vi "PrototypeV2_control.vi"() -> ()   [LabVIEW 2019]
uses:
  00d467ad-0018-435b-b1c4-002e486b128f.vi
  2e8d34c2-00e2-46f1-99d0-d57288b70d8f.vi
  0f690846-c94a-4028-9fe1-d10e28cf598c.vi
  4854abb9-ccb6-456c-8c0d-1df9cc9317d1.vi
  <vilib>/Instr/_visa.llb/VISA Configure Serial Port (Instr).vi
  globals.vi
  <vilib>/Utility/file.llb/Read Delimited Spreadsheet (DBL).vi
panel:
  in  "Control SAS":bool
  in  "Control ELO":bool
  in  "UVP OVP BAT2":bool=TRUE
  in  "UVP OVP BAT1":bool=TRUE
  in  "ELO file":path=path "C:/repositories/bdc_controller/hex_logger/source_code/0.5A.csv"
  in  "ELO VISA":refnum<visa-resource-name>="USB0::0x0B3E::0x1019::YL002399::INSTR"
  in  "Orbits":i32=4
  out "Orbital period (s)":dbl
  out "elapsed time":dbl
  in  "SAS file":path=path "C:/repositories/bdc_controller/hex_logger/source_code/SAS_off.csv"
  in  "SAS VISA":refnum<visa-resource-name>="USB0::0x0957::0x1107::MY54001612::INSTR"
  out "CONV2":cluster{u16, u16, i16}(graph)
  out "converter2 file":path
  out "controller file":path
  out "converter1 file":path
  in  "CONVERTER 2 PORT":refnum<visa-resource-name>="COM5"
  out "sync":bool
  in  "CONVERTER 1 PORT":refnum<visa-resource-name>="COM4"
  out "sync":bool
  out "CONV1":cluster{u16, u16, i16}(graph)
  out "3.3V REG":cluster{u16, u16}(graph)
  out "5V REG":cluster{u16, u16}(graph)
  out "BUS":cluster{u16, u16, u16}(graph)
  in  "project name":string
  in  "CONTROL":bool
  in  "CONTROLLER PORT":refnum<visa-resource-name>="COM3"
  out "sync":bool
  in  "STOP":bool
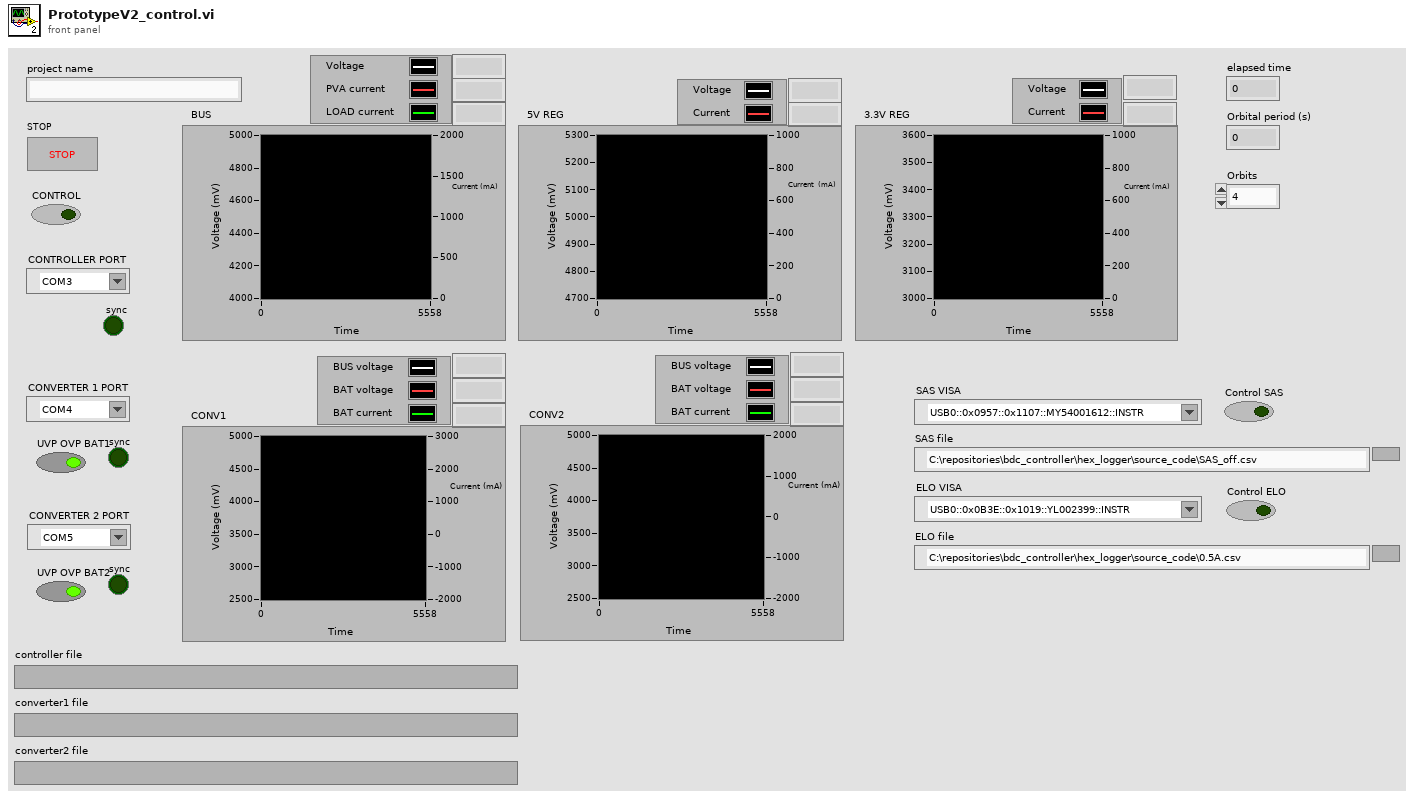
[diagram p1: front panel]
types:
  T1 = cluster{u16, u16, u16, u16, u16, u16, u16, u16, u16}
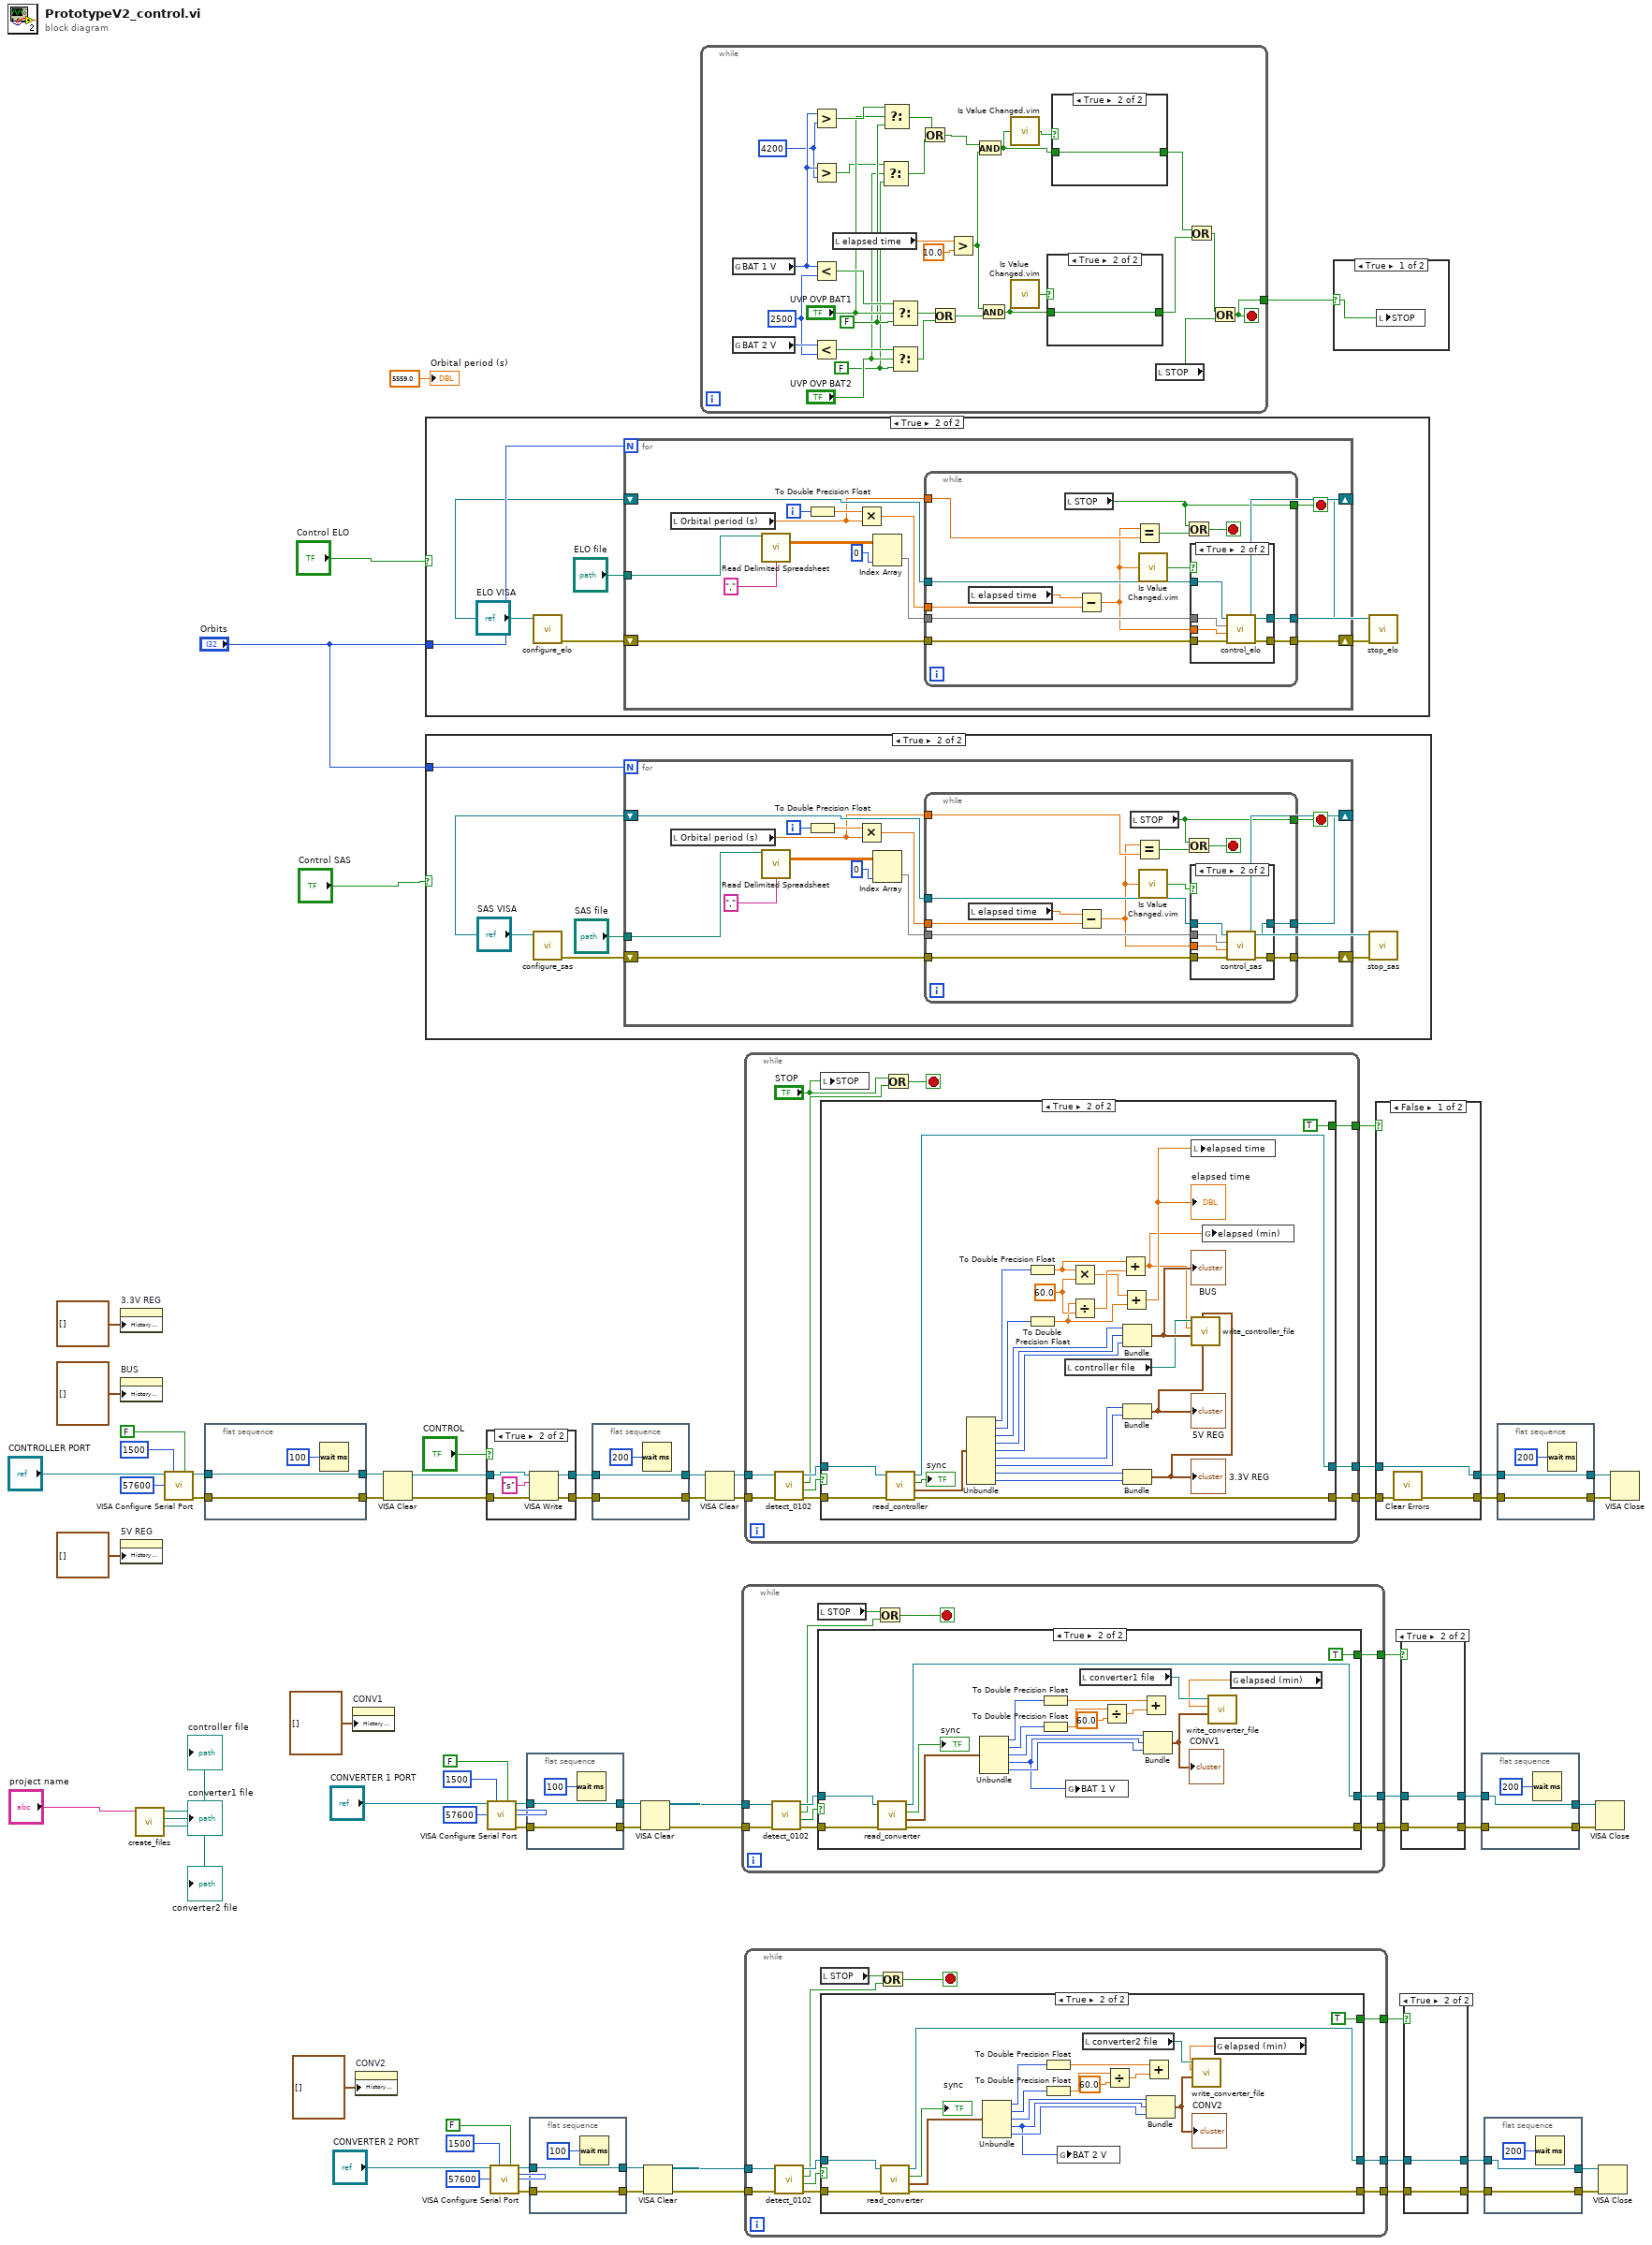
[diagram p0: block diagram]
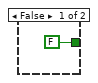
[diagram p7: hidden frame]
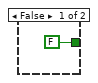
[diagram p8: hidden frame]
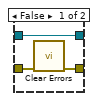
[diagram p9: hidden frame]
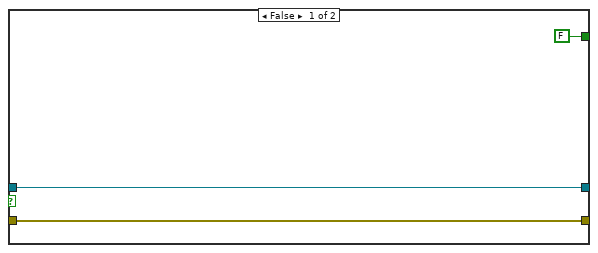
[diagram p10: hidden frame]
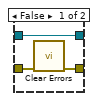
[diagram p11: hidden frame]
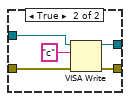
[diagram p12: hidden frame]
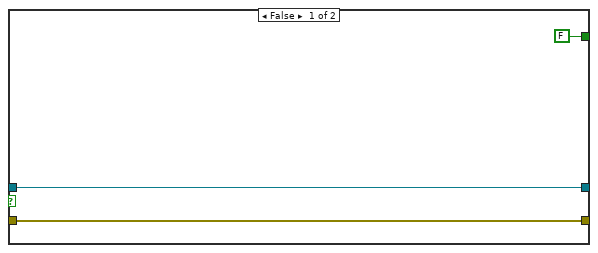
[diagram p13: hidden frame]
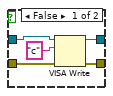
[diagram p14: hidden frame]
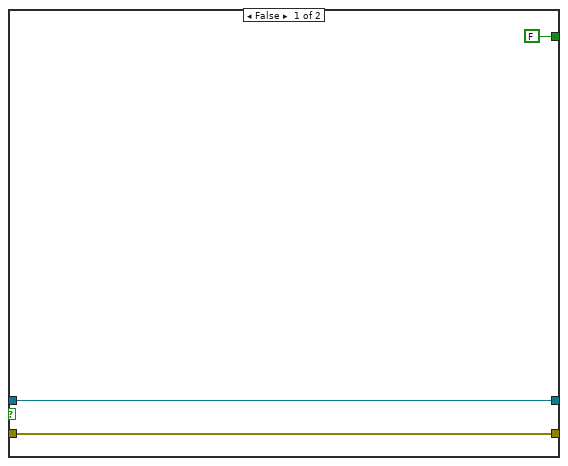
[diagram p15: hidden frame]
diagram:
  n1 = property on="3.3V REG" class="WFChart (strict)"("History Data"=cluster{dbl, dbl}[] []) -> ()  [unwired: 2 in, 2 out]
  n2 = property on="BUS" class="WFChart (strict)"("History Data"=cluster{dbl, dbl, dbl}[] []) -> ()  [unwired: 2 in, 2 out]
  n3 = property on="5V REG" class="WFChart (strict)"("History Data"=cluster{dbl, dbl}[] []) -> ()  [unwired: 2 in, 2 out]
  n4 = call "create_files.vi"("project name"="project name") -> ("converter2"=→"converter2 file":path, "converter1"=→"converter1 file":path, "controller"=→"controller file":path)  [unwired: 8 in]
  n5 = call-poly "VISA Configure Serial Port"("VISA resource name"="CONTROLLER PORT", "timeout (10sec)"=u32 1500, "Enable Termination\nChar (T)"=FALSE ("Enable Termination\nChar (T)"), "baud rate (9600)"=u32 57600) -> ("VISA resource name out"=w69:refnum<visa-resource-name>, "error out"=w68:errorcluster)  [unwired: 10 in]
  n6 = flat-sequence {
    tunnel: w68 -> [w74]
    tunnel: [w74] -> w67
    tunnel: [w73] -> w66
    tunnel: w69 -> [w73]
    frame #0 {
      n7 = Wait (ms)(milliseconds to wait=u32 100) -> ()  [unwired: 1 out]
    }
  }
  n8 = property on="CONV1" class="WFChart (strict)"("History Data"=cluster{dbl, dbl, dbl}[] []) -> ()  [unwired: 2 in, 2 out]
  n9 = property on="CONV2" class="WFChart (strict)"("History Data"=cluster{dbl, dbl, dbl}[] []) -> ()  [unwired: 2 in, 2 out]
  n10 = VISA Clear(VISA resource name=w66, error in (no error)=w67) -> (VISA resource name out=w65:refnum<visa-resource-name>, error out=w64:errorcluster)
  n11 = case shown="True" "Control ELO" {
    tunnel: "Orbits" -> [_ w81]
    frame False {
    }
    frame True {
      n12 = call "configure_elo.vi"("VISA Refnum in"="ELO VISA") -> ("error out"=w78:errorcluster, "VISA Refnum out"=w79:refnum<visa-resource-name>)  [unwired: 8 in, 1 out]
      n13 = for {
        N: w81 -> [_]
        shift-right: [w94] -> w77
        shift-left: w79 -> [w96]
        shift-right: [w93] -> w76
        shift-left: w78 -> [w95]
        tunnel: "ELO file" -> [w85]
        i -> [w91]
        stop <- w83 stop-if-true
        n14 = local read "Orbital period (s)"() -> (w89:dbl)
        n15 = call-poly <vilib>:"Read Delimited Spreadsheet.vi"("file path (dialog if empty)"=w85, "delimiter (\\t)"="," ("delimiter (\\t)")) -> ("all rows"=w88:dbl[][])  [unwired: 8 in, 5 out]
        n16 = To Double Precision Float(number=w91) -> (double precision float=w92:dbl)
        n17 = Multiply(x=w92, y=w89) -> (x*y=w90:dbl)
        n18 = Index Array(array=w88, index (col)=0 ("disabled index (col)")) -> (element=w84:dbl[])  [unwired: 1 in]
        n19 = while {
          tunnel: w96 -> [w109]
          tunnel: w95 -> [w108]
          tunnel: w84 -> [w107]
          tunnel: [w105] -> w94
          tunnel: [w104] -> w93
          tunnel: w90 -> [w103]
          tunnel: w89 -> [w101]
          tunnel: [w97] -> w83
          stop <- w98 stop-if-true
          n20 = local read "elapsed time"() -> (w102:dbl)
          n21 = local read "STOP"() -> (w97:bool)
          n22 = Subtract(x=w102, y=w103) -> (x-y=w100:dbl)
          n23 = Equal?(x=w100, y=w101) -> (x = y?=w99:bool)
          n24 = call "Is Value Changed.vim"("value"=w100) -> ("changed or first call?"=w106:bool)
          n25 = Or(x=w97, y=w99) -> (x .or. y?=w98:bool)
          n26 = case shown="True" w106 {
            tunnel: w109 -> [w111 w117]
            tunnel: w108 -> [w110 w116]
            tunnel: w100 -> [_ w115]
            tunnel: w107 -> [_ w114]
            tunnel: [w111 w113] -> w105
            tunnel: [w110 w112] -> w104
            frame False {
            }
            frame True {
              n27 = call "control_elo.vi"("error in (no error)"=w116, "Numeric"=w115, "all rows"=w114, "VISA Refnum in"=w117) -> ("error out"=w112:errorcluster, "VISA Refnum out"=w113:refnum<visa-resource-name>)  [unwired: 6 in]
            }
          }
        }
      }
      n28 = call "stop_elo.vi"("error in (no error)"=w76, "VISA Refnum in"=w77) -> ()  [unwired: 10 in]
    }
  }
  n29 = case shown="True" "Control SAS" {
    tunnel: "Orbits" -> [_ w118]
    frame False {
    }
    frame True {
      n30 = call "configure_sas.vi"("VISA Refnum in"="SAS VISA") -> ("error out"=w122:errorcluster, "VISA Refnum out"=w123:refnum<visa-resource-name>)  [unwired: 7 in]
      n31 = for {
        N: w118 -> [_]
        shift-right: [w136] -> w121
        shift-left: w123 -> [w138]
        shift-right: [w135] -> w120
        shift-left: w122 -> [w137]
        tunnel: "SAS file" -> [w127]
        i -> [w133]
        stop <- w125 stop-if-true
        n32 = local read "Orbital period (s)"() -> (w131:dbl)
        n33 = call-poly <vilib>:"Read Delimited Spreadsheet.vi"("file path (dialog if empty)"=w127, "delimiter (\\t)"="," ("delimiter (\\t)")) -> ("all rows"=w130:dbl[][])  [unwired: 8 in, 5 out]
        n34 = To Double Precision Float(number=w133) -> (double precision float=w134:dbl)
        n35 = Multiply(x=w134, y=w131) -> (x*y=w132:dbl)
        n36 = Index Array(array=w130, index (col)=0 ("disabled index (col)")) -> (element=w126:dbl[])  [unwired: 1 in]
        n37 = while {
          tunnel: w138 -> [w151]
          tunnel: w137 -> [w150]
          tunnel: w126 -> [w149]
          tunnel: [w147] -> w136
          tunnel: [w146] -> w135
          tunnel: w132 -> [w145]
          tunnel: w131 -> [w143]
          tunnel: [w141] -> w125
          stop <- w139 stop-if-true
          n38 = local read "elapsed time"() -> (w144:dbl)
          n39 = Subtract(x=w144, y=w145) -> (x-y=w142:dbl)
          n40 = local read "STOP"() -> (w141:bool)
          n41 = Equal?(x=w142, y=w143) -> (x = y?=w140:bool)
          n42 = call "Is Value Changed.vim"("value"=w142) -> ("changed or first call?"=w148:bool)
          n43 = Or(x=w141, y=w140) -> (x .or. y?=w139:bool)
          n44 = case shown="True" w148 {
            tunnel: w151 -> [w153 w158]
            tunnel: w150 -> [w152 w157]
            tunnel: w142 -> [_ w155]
            tunnel: w149 -> [_ w156]
            tunnel: [w153 w154] -> w147
            tunnel: [w152 w159] -> w146
            frame False {
            }
            frame True {
              n45 = call "control_sas.vi"("error in (no error)"=w157, "Numeric"=w155, "all rows"=w156, "VISA Refnum in"=w158) -> ("error out"=w159:errorcluster, "VISA Refnum out"=w154:refnum<visa-resource-name>)  [unwired: 6 in]
            }
          }
        }
      }
      n46 = call "stop_sas.vi"("error in (no error)"=w120, "VISA Refnum in"=w121) -> ()  [unwired: 10 in]
    }
  }
  n47 = case shown="True" "CONTROL" {
    tunnel: w65 -> [w163 w169]
    tunnel: [w161 w168] -> w62
    tunnel: w64 -> [w162 w167]
    tunnel: [w160 w166] -> w61
    frame False {
      n48 = VISA Write(VISA resource name=w163, write buffer="c", error in (no error)=w162) -> (VISA resource name out=w161:refnum<visa-resource-name>, error out=w160:errorcluster)  [unwired: 1 out]
    }
    frame True {
      n49 = VISA Write(VISA resource name=w169, write buffer="s", error in (no error)=w167) -> (VISA resource name out=w168:refnum<visa-resource-name>, error out=w166:errorcluster)  [unwired: 1 out]
    }
  }
  n50 = call-poly "VISA Configure Serial Port"("VISA resource name"="CONVERTER 1 PORT", "timeout (10sec)"=u32 1500, "Enable Termination\nChar (T)"=FALSE ("Enable Termination\nChar (T)"), "baud rate (9600)"=u32 57600) -> ("VISA resource name out"=w44:refnum<visa-resource-name>, "error out"=w43:errorcluster)  [unwired: 10 in]
  n51 = call-poly "VISA Configure Serial Port"("VISA resource name"="CONVERTER 2 PORT", "timeout (10sec)"=u32 1500, "Enable Termination\nChar (T)"=FALSE ("Enable Termination\nChar (T)"), "baud rate (9600)"=u32 57600) -> ("VISA resource name out"=w21:refnum<visa-resource-name>, "error out"=w20:errorcluster)  [unwired: 10 in]
  n52 = flat-sequence {
    tunnel: w43 -> [w171]
    tunnel: [w171] -> w42
    tunnel: [w170] -> w41
    tunnel: w44 -> [w170]
    frame #0 {
      n53 = Wait (ms)(milliseconds to wait=u32 100) -> ()  [unwired: 1 out]
    }
  }
  n54 = flat-sequence {
    tunnel: w20 -> [w174]
    tunnel: [w174] -> w19
    tunnel: [w173] -> w18
    tunnel: w21 -> [w173]
    frame #0 {
      n55 = Wait (ms)(milliseconds to wait=u32 100) -> ()  [unwired: 1 out]
    }
  }
  n56 = flat-sequence {
    tunnel: w61 -> [w177]
    tunnel: [w177] -> w58
    tunnel: [w176] -> w60
    tunnel: w62 -> [w176]
    frame #0 {
      n57 = Wait (ms)(milliseconds to wait=u32 200) -> ()  [unwired: 1 out]
    }
  }
  n58 = VISA Clear(VISA resource name=w41, error in (no error)=w42) -> (VISA resource name out=w26:refnum<visa-resource-name>, error out=w25:errorcluster)
  n59 = VISA Clear(VISA resource name=w18, error in (no error)=w19) -> (VISA resource name out=w9:refnum<visa-resource-name>, error out=w8:errorcluster)
  n60 = while {
    tunnel: [w179] -> w1
    stop <- w179 stop-if-true
    w195 = u16 4200 ("y")
    w189 = FALSE ("f")
    w192 = FALSE ("f")
    w207 = u16 2500 ("y")
    n61 = global read "globals.vi" "BAT 1 V"() -> (w196:u16)
    n62 = global read "globals.vi" "BAT 2 V"() -> (w208:u16)
    n63 = Greater?(x=w196, y=w195) -> (0:w194:bool)
    n64 = Greater?(x=w196, y=w195) -> (0:w191:bool)
    n65 = Less?(x=w196, y=w207) -> (x < y?=w206:bool)
    n66 = Less?(x=w208, y=w207) -> (x < y?=w205:bool)
    n67 = local read "elapsed time"() -> (w201:dbl)
    n68 = Select(t=w191, s="UVP OVP BAT2", f=w189) -> (s? t:f=w187:bool)
    n69 = Select(t=w194, s="UVP OVP BAT1", f=w192) -> (s? t:f=w188:bool)
    n70 = Select(t=w206, s="UVP OVP BAT1", f=w192) -> (s? t:f=w204:bool)
    n71 = Select(t=w205, s="UVP OVP BAT2", f=w189) -> (s? t:f=w203:bool)
    n72 = Or(x=w188, y=w187) -> (x .or. y?=w185:bool)
    n73 = Or(x=w204, y=w203) -> (x .or. y?=w199:bool)
    n74 = Greater?(x=w201, y=10.0) -> (0:w186:bool)
    n75 = And(x=w185, y=w186) -> (x .and. y?=w183:bool)
    n76 = And(x=w186, y=w199) -> (x .and. y?=w198:bool)
    n77 = call "Is Value Changed.vim"("value"=w183) -> ("changed or first call?"=w184:bool)
    n78 = call "Is Value Changed.vim"("value"=w198) -> ("changed or first call?"=w202:bool)
    n79 = case shown="True" w202 {
      tunnel: [FALSE w212] -> w181
      tunnel: w198 -> [_ w212]
      frame False {
      }
      frame True {
      }
    }
    n80 = case shown="True" w184 {
      tunnel: [FALSE w210] -> w182
      tunnel: w183 -> [_ w210]
      frame False {
      }
      frame True {
      }
    }
    n81 = local read "STOP"() -> (w197:bool)
    n82 = Or(x=w182, y=w181) -> (x .or. y?=w180:bool)
    n83 = Or(x=w180, y=w197) -> (x .or. y?=w179:bool)
  }
  n84 = VISA Clear(VISA resource name=w60, error in (no error)=w58) -> (VISA resource name out=w59:refnum<visa-resource-name>, error out=w57:errorcluster)
  n85 = while {
    tunnel: w25 -> [w218]
    tunnel: [w222] -> w32
    tunnel: [w223] -> w33
    tunnel: w26 -> [w219]
    tunnel: [w220] -> w31
    stop <- w221 stop-if-true
    n86 = call "detect_0102.vi"("error in (no error)"=w218, "VISA Refnum in"=w219) -> ("error out"=w216:errorcluster, "RECEIVED"=w214:bool, "NOT RECEIVED"=w215:bool, "VISA Refnum out"=w217:refnum<visa-resource-name>)  [unwired: 6 in]
    n87 = local read "STOP"() -> (w213:bool)
    n88 = case shown="True" w214 {
      tunnel: w217 -> [w226 w238]
      tunnel: w216 -> [w225 w233]
      tunnel: [w226 w234] -> w223
      tunnel: [w225 w237] -> w222
      tunnel: [FALSE TRUE] -> w220
      frame False {
      }
      frame True {
        n89 = call "read_converter.vi"("error in (no error)"=w233, "VISA Refnum in"=w238) -> ("error out"=w237:errorcluster, "Types?"=w235:cluster{u16, u16, u16, u16, i16}, "sync"=→"sync":bool, "VISA Refnum out"=w234:refnum<visa-resource-name>)  [unwired: 6 in]
        n90 = Unbundle(w235) -> (w245:u16, w244:u16, w230:u16, w228:u16, w229:i16)
        n91 = To Double Precision Float(number=w245) -> (double precision float=w241:dbl)
        n92 = To Double Precision Float(number=w244) -> (double precision float=w242:dbl)
        n93 = global write "globals.vi" "BAT 1 V"(w228) -> ()
        n94 = local read "converter1 file"() -> (w231:path)
        n95 = Divide(x=w242, y=60.0) -> (x/y=w240:dbl)
        n96 = Add(x=w241, y=w240) -> ()  [unwired: 1 out]
        n97 = Bundle(w230, w228, w229) -> (w232:cluster{u16, u16, i16})  [unwired: 1 in]
        "CONV1" <- w232
        n98 = global read "globals.vi" "elapsed (min)"() -> (w227:dbl)
        n99 = call "write_converter_file.vi"("CONVERTER"=w232, "minutes"=w227, "converter file"=w231) -> ()  [unwired: 9 in]
      }
    }
    n100 = Or(x=w213, y=w215) -> (x .or. y?=w221:bool)
  }
  n101 = while {
    tunnel: w57 -> [w254]
    tunnel: [w251] -> w55
    tunnel: [w252] -> w56
    tunnel: w59 -> [w253]
    tunnel: [w247] -> w39
    stop <- w250 stop-if-true
    n102 = call "detect_0102.vi"("error in (no error)"=w254, "VISA Refnum in"=w253) -> ("error out"=w255:errorcluster, "RECEIVED"=w248:bool, "NOT RECEIVED"=w249:bool, "VISA Refnum out"=w256:refnum<visa-resource-name>)  [unwired: 6 in]
    n103 = local write "STOP"("STOP") -> ()
    n104 = case shown="True" w248 {
      tunnel: w256 -> [w259 w286]
      tunnel: w255 -> [w258 w285]
      tunnel: [w259 w280] -> w252
      tunnel: [w258 w279] -> w251
      tunnel: [FALSE TRUE] -> w247
      frame False {
      }
      frame True {
        w271 = 60.0 ("y")
        n105 = call "read_controller.vi"("error in (no error)"=w285, "VISA Refnum in"=w286) -> ("error out"=w279:errorcluster, "Type?"=w284:T1, "sync"=→"sync":bool, "VISA Refnum out"=w280:refnum<visa-resource-name>)  [unwired: 6 in]
        n106 = Unbundle(w284) -> (w283:u16, w282:u16, w267:u16, w266:u16, w265:u16, w264:u16, w263:u16, w262:u16, w261:u16)
        n107 = To Double Precision Float(number=w283) -> (double precision float=w272:dbl)
        n108 = To Double Precision Float(number=w282) -> (double precision float=w269:dbl)
        n109 = local read "controller file"() -> (w275:path)
        n110 = Multiply(x=w272, y=w271) -> (x*y=w270:dbl)
        n111 = Divide(x=w269, y=w271) -> (x/y=w281:dbl)
        n112 = Add(x=w272, y=w281) -> (x+y=w260:dbl)
        n113 = Add(x=w270, y=w269) -> (x+y=w268:dbl)
        "elapsed time" <- w268
        n114 = Bundle(w267, w266, w265) -> (w276:cluster{u16, u16, u16})  [unwired: 1 in]
        "BUS" <- w276
        n115 = Bundle(w264, w263) -> (w274:cluster{u16, u16})  [unwired: 1 in]
        "5V REG" <- w274
        n116 = Bundle(w262, w261) -> (w273:cluster{u16, u16})  [unwired: 1 in]
        "3.3V REG" <- w273
        n117 = local write "elapsed time"(w268) -> ()
        n118 = call "write_controller_file.vi"("5V reg"=w274, "3.3V reg"=w273, "BUS"=w276, "minutes"=w260, "controller file"=w275) -> ()  [unwired: 7 in]
        n119 = global write "globals.vi" "elapsed (min)"(w260) -> ()
      }
    }
    n120 = Or(x="STOP", y=w249) -> (x .or. y?=w250:bool)
  }
  n121 = while {
    tunnel: w8 -> [w292]
    tunnel: [w296] -> w11
    tunnel: [w297] -> w12
    tunnel: w9 -> [w293]
    tunnel: [w294] -> w10
    stop <- w295 stop-if-true
    n122 = call "detect_0102.vi"("error in (no error)"=w292, "VISA Refnum in"=w293) -> ("error out"=w290:errorcluster, "RECEIVED"=w288:bool, "NOT RECEIVED"=w289:bool, "VISA Refnum out"=w291:refnum<visa-resource-name>)  [unwired: 6 in]
    n123 = local read "STOP"() -> (w287:bool)
    n124 = case shown="True" w288 {
      tunnel: w291 -> [w300 w312]
      tunnel: w290 -> [w299 w308]
      tunnel: [w300 w309] -> w297
      tunnel: [w299 w311] -> w296
      tunnel: [FALSE TRUE] -> w294
      frame False {
      }
      frame True {
        n125 = call "read_converter.vi"("error in (no error)"=w308, "VISA Refnum in"=w312) -> ("error out"=w311:errorcluster, "Types?"=w310:cluster{u16, u16, u16, u16, i16}, "sync"=→"sync":bool, "VISA Refnum out"=w309:refnum<visa-resource-name>)  [unwired: 6 in]
        n126 = Unbundle(w310) -> (w319:u16, w318:u16, w304:u16, w302:u16, w303:i16)
        n127 = To Double Precision Float(number=w319) -> (double precision float=w315:dbl)
        n128 = To Double Precision Float(number=w318) -> (double precision float=w316:dbl)
        n129 = global write "globals.vi" "BAT 2 V"(w302) -> ()
        n130 = local read "converter2 file"() -> (w305:path)
        n131 = Divide(x=w316, y=60.0) -> (x/y=w314:dbl)
        n132 = Add(x=w315, y=w314) -> ()  [unwired: 1 out]
        n133 = Bundle(w304, w302, w303) -> (w306:cluster{u16, u16, i16})  [unwired: 1 in]
        "CONV2" <- w306
        n134 = global read "globals.vi" "elapsed (min)"() -> (w301:dbl)
        n135 = call "write_converter_file.vi"("CONVERTER"=w306, "minutes"=w301, "converter file"=w305) -> ()  [unwired: 9 in]
      }
    }
    n136 = Or(x=w287, y=w289) -> (x .or. y?=w295:bool)
  }
  n137 = case shown="True" w1 {
    selector: w1 -> [w320 _]
    frame True {
      n138 = local write "STOP"(w320) -> ()
    }
    frame False {
    }
  }
  n139 = case shown="False" w39 {
    tunnel: w56 -> [w323 w327]
    tunnel: w55 -> [w322 w326]
    tunnel: [w323 w325] -> w54
    tunnel: [w321 w324] -> w53
    frame False {
      n140 = call <vilib>:"Clear Errors.vi"("error in (no error)"=w322) -> ("error out"=w321:errorcluster)  [unwired: 5 in, 1 out]
    }
    frame True {
      n141 = VISA Write(VISA resource name=w327, write buffer="c", error in (no error)=w326) -> (VISA resource name out=w325:refnum<visa-resource-name>, error out=w324:errorcluster)  [unwired: 1 out]
    }
  }
  n142 = case shown="True" w31 {
    tunnel: w33 -> [w331 w333]
    tunnel: w32 -> [w330 w332]
    tunnel: [w331 w333] -> w37
    tunnel: [w329 w332] -> w36
    frame False {
      n143 = call <vilib>:"Clear Errors.vi"("error in (no error)"=w330) -> ("error out"=w329:errorcluster)  [unwired: 5 in, 1 out]
    }
    frame True {
    }
  }
  n144 = case shown="True" w10 {
    tunnel: w12 -> [w336 w338]
    tunnel: w11 -> [w335 w337]
    tunnel: [w336 w338] -> w16
    tunnel: [w334 w337] -> w15
    frame False {
      n145 = call <vilib>:"Clear Errors.vi"("error in (no error)"=w335) -> ("error out"=w334:errorcluster)  [unwired: 5 in, 1 out]
    }
    frame True {
    }
  }
  n146 = flat-sequence {
    tunnel: w36 -> [w340]
    tunnel: [w340] -> w35
    tunnel: [w339] -> w34
    tunnel: w37 -> [w339]
    frame #0 {
      n147 = Wait (ms)(milliseconds to wait=u32 200) -> ()  [unwired: 1 out]
    }
  }
  n148 = flat-sequence {
    tunnel: w15 -> [w343]
    tunnel: [w343] -> w14
    tunnel: [w342] -> w13
    tunnel: w16 -> [w342]
    frame #0 {
      n149 = Wait (ms)(milliseconds to wait=u32 200) -> ()  [unwired: 1 out]
    }
  }
  n150 = flat-sequence {
    tunnel: w53 -> [w346]
    tunnel: [w346] -> w52
    tunnel: [w345] -> w51
    tunnel: w54 -> [w345]
    frame #0 {
      n151 = Wait (ms)(milliseconds to wait=u32 200) -> ()  [unwired: 1 out]
    }
  }
  n152 = VISA Close(VISA resource name=w34, error in (no error)=w35) -> ()  [unwired: 1 out]
  n153 = VISA Close(VISA resource name=w13, error in (no error)=w14) -> ()  [unwired: 1 out]
  n154 = VISA Close(VISA resource name=w51, error in (no error)=w52) -> ()  [unwired: 1 out]
  "Orbital period (s)" <- 5559.0 ("Orbital period")
